vi "Response queue.vi"(3 "Action":T2(ring), 4 "Prompt of item possibly in queue":string, 5 "New item":T1) -> (0 "Item present (& removed)?":bool, 1 "Response":bool)   [LabVIEW 2011]
uses:
  Response queue item.ctl
panel:
  out "Queue":T1[](array[typedef])
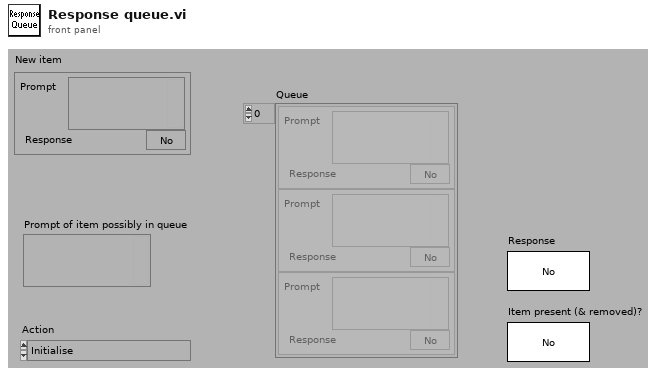
[diagram p1: front panel]
types:
  T1 = typedef "Response queue item.ctl" = cluster{"Prompt":string, "Response":bool}
  T2 = enum16{"Initialise", "Add", "Check for response & remove"}
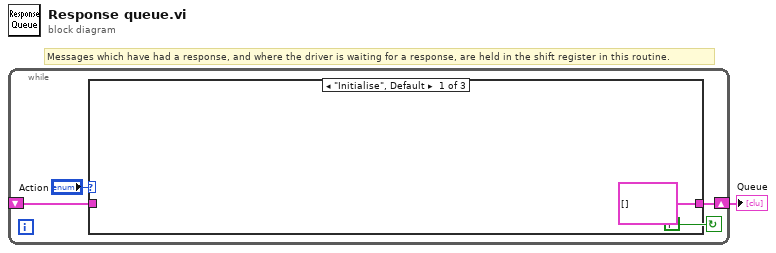
[diagram p0: block diagram]
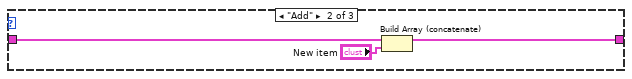
[diagram p2: hidden frame]
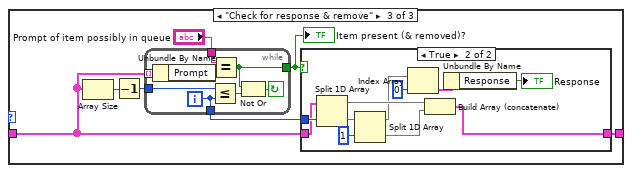
[diagram p3: hidden frame]
diagram:
  # "Messages which have had a response, and where the driver is waiting for a response, are held in the shift register in this routine."
  n1 = while {
    shift-left: _ -> [w3]
    shift-right: [w4] -> w1
    stop <- FALSE continue-if-true
    n2 = case shown="\"Initialise\", Default" "Action" {
      tunnel: [T1[] [] ("Queue in") w7 w12] -> w4
      tunnel: w3 -> [_ w9 w16]
      frame "Initialise", Default {
      }
      frame "Add" {
        n3 = Build Array (concatenate)(w9, "New item") -> (w7:T1[])
      }
      frame "Check for response & remove" {
        n4 = Array Size(array=w16) -> (size(s)=w15:i32)
        n5 = Decrement(x=w15) -> (x-1=w14:i32)
        n6 = while {
          tunnel: [w17] -> w10
          tunnel: "Prompt of item possibly in queue" -> [w19]
          tunnel: [w21] -> w13
          tunnel: w16 -> [w24] mode=indexing
          tunnel: w14 -> [w23]
          i -> [w21]
          stop <- w22 continue-if-true
          n7 = Unbundle By Name(w24) -> ("Prompt"=w18:string)
          n8 = Less Or Equal?(x=w23, y=w21) -> (x <= y?=w20:bool)
          n9 = Equal?(x=w19, y=w18) -> (x = y?=w17:bool)
          n10 = Not Or(1:w20, 2:w17) -> (0:w22:bool)
        }
        "Item present (& removed)?" <- w10
        n11 = case shown="True" w10 {
          tunnel: w13 -> [_ w36]
          tunnel: w16 -> [w25 w35]
          tunnel: [w25 w30] -> w12
          frame False {
          }
          frame True {
            n12 = Split 1D Array(array=w35, index=w36) -> (first subarray=w32:T1[], second subarray=w34:T1[])
            n13 = Split 1D Array(array=w34, index=1) -> (first subarray=w29:T1[], second subarray=w31:T1[])
            n14 = Index Array(array=w29, index=0 ("Index")) -> (element=w27:T1)
            n15 = Build Array (concatenate)(w32, w31) -> (w30:T1[])
            n16 = Unbundle By Name(w27) -> ("Response"=→"Response":bool)
          }
        }
      }
    }
  }
  "Queue" <- w1
